vi "RT_Main.vi"() -> (2 "running":bool)   [LabVIEW 2018]
uses:
  <vilib>/FPGAPlugInAG/myRIO-1900/niLvFpga_Open_myRIO-1900.vi
  <vilib>/rvi/interface/common/dynamic/niFpgaDynamicAddResources.vi
  <vilib>/Utility/error.llb/Error Cluster From Error Code.vi
  <vilib>/rvi/errors/niLvFpgaAdjustHostInterfaceError.vi
  <vilib>/rvi/interface/common/niFpgaWaitOnOcc.vi
  <vilib>/FPGAPlugInAG/Dynamic/niLvFpga_Close_Dynamic.vi
  <vilib>/rvi/interface/nirviOpenFPGA/nirviOpenFPGA.xnode
  FPGA Bitfiles/FPGAPLL_FPGATarget_FPGAMain_V3ImA1lHnbc.lvbitx
  FPGA_Main.vi
  <vilib>/rvi/interface/nirviReadWriteControl/nirviReadWriteControl.xnode
  <vilib>/rvi/interface/nirviMethod/nirviMethod.xnode
  <vilib>/rvi/interface/nirviCloseFPGA/nirviCloseFPGA.xnode
  <vilib>/rvi/errors/niLvFpgaMergeErrorWithErrorCode.vi
  <vilib>/FPGAPlugInAG/Dynamic/niLvFpga_ReadFifo_Dynamic.vi
  <vilib>/FPGAPlugInAG/Dynamic/niLvFpga_ConfigureFifo_Dynamic.vi
  <vilib>/FPGAPlugInAG/Dynamic/niLvFpga_StartFifo_Dynamic.vi
  NiFpgaLv.dll
  <vilib>/rvi/interface/Simulation/niFpgaSimulationCallBeginRW.vi
panel:
  out "size(s)":i32
  out "error fifo\nread data":errorcluster
  out "#element left":u32
  out "#elements":u32
  out "error fifo start":errorcluster
  out "error fifo \ncheck #E":errorcluster
  out "error ref":errorcluster
  out "error closing":errorcluster
  out "error fifo config":errorcluster
  out "Actual Depth":u32
  # "RT Main"
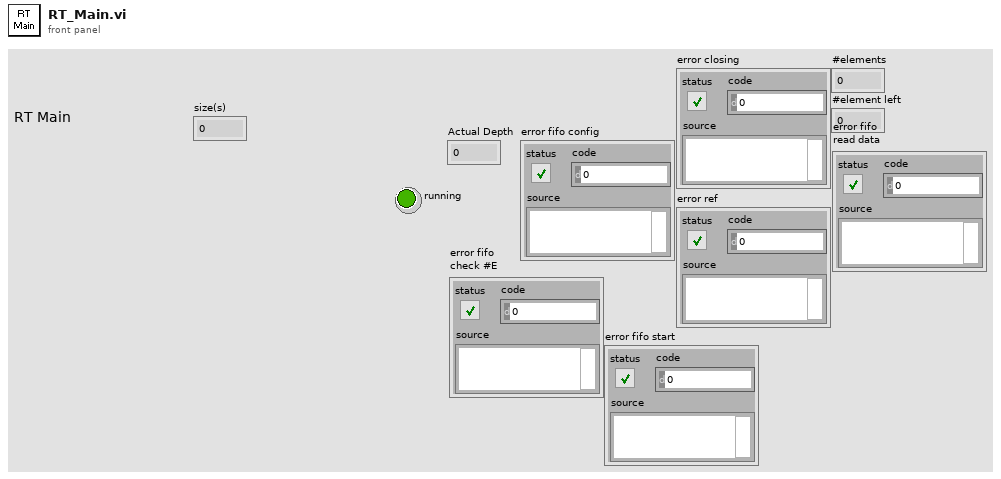
[diagram p1: front panel]
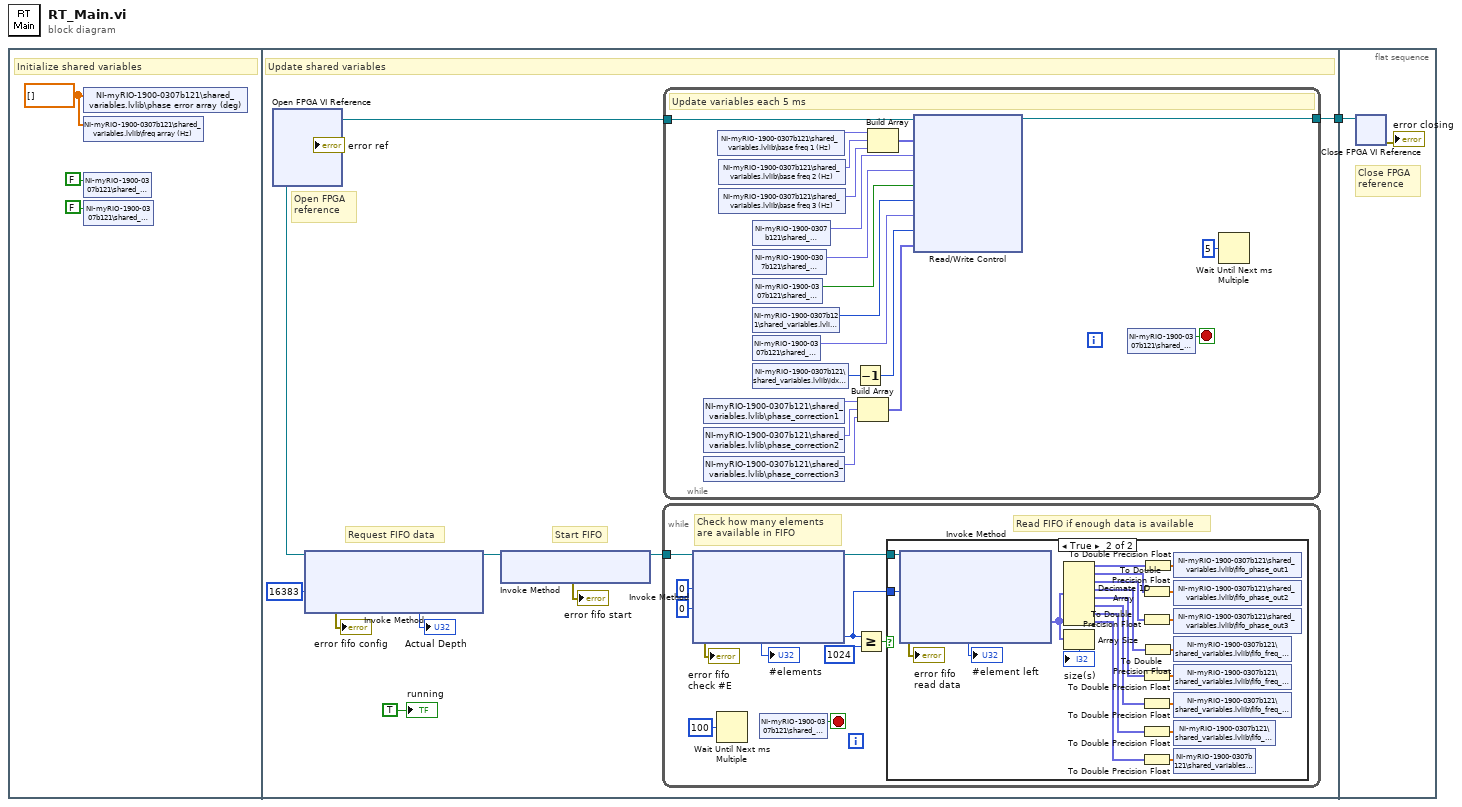
[diagram p0: block diagram]
diagram:
  n1 = flat-sequence {
    tunnel: [w13] -> w1
    tunnel: w1 -> [w67]
    frame #0 {
      w2 = dbl[] [] ("phase error array (deg)")
      # "Initialize shared variables"
      n2 = shared-variable "NI-myRIO-1900-0307b121\\shared_variables.lvlib\\phase error array (deg)"(w2) -> ()  [unwired: 1 in, 1 out]
      n3 = shared-variable "NI-myRIO-1900-0307b121\\shared_variables.lvlib\\freq array (Hz)"(w2) -> ()  [unwired: 1 in, 1 out]
      n4 = shared-variable "NI-myRIO-1900-0307b121\\shared_variables.lvlib\\stop"(FALSE ("stop")) -> ()  [unwired: 1 in, 1 out]
      n5 = shared-variable "NI-myRIO-1900-0307b121\\shared_variables.lvlib\\reset"(FALSE ("reset")) -> ()  [unwired: 1 in, 1 out]
    }
    frame #1 {
      # "Start FIFO"
      # "Request FIFO data"
      # "Open FPGA\nreference"
      # "Update shared variables"
      n6 = xnode "Open FPGA VI Reference"() -> ("FPGA VI Reference Out"=w12:refnum<k20>, "error out"=→"error ref":errorcluster)  [unwired: 2 in]
      n7 = xnode "Invoke Method"("FPGA VI Reference In"=w12, "Requested Depth"=u32 16383) -> ("FPGA VI Reference Out"=w7:refnum<k20>, "error out"=→"error fifo config":errorcluster, "Actual Depth"=→"Actual Depth":u32)  [unwired: 1 in]
      n8 = xnode "Invoke Method"("FPGA VI Reference In"=w7) -> ("FPGA VI Reference Out"=w5:refnum<k20>, "error out"=→"error fifo start":errorcluster)  [unwired: 1 in]
      n9 = while {
        tunnel: w5 -> [w23]
        stop <- w24 stop-if-true
        # "Read FIFO if enough data is available"
        # "Check how many elements\nare available in FIFO"
        n10 = xnode "Invoke Method"("FPGA VI Reference In"=w23, "Number of Elements"=u32 0, "Timeout (ms)"=0) -> ("FPGA VI Reference Out"=w18:refnum<k20>, "error out"=→"error fifo \ncheck #E":errorcluster, "Elements Remaining"=w16:u32)  [unwired: 1 in, 1 out]
        "#elements" <- w16
        n11 = Wait Until Next ms Multiple(millisecond multiple=u32 100) -> ()  [unwired: 1 out]
        n12 = shared-variable "NI-myRIO-1900-0307b121\\shared_variables.lvlib\\stop"() -> (w24:bool)  [unwired: 1 in, 1 out]
        n13 = Greater Or Equal?(x=w16, y=u32 1024) -> (x >= y?=w15:bool)
        n14 = case shown="True" w15 {
          tunnel: w18 -> [_ w46]
          tunnel: w16 -> [_ w41]
          frame False {
          }
          frame True {
            n15 = xnode "Invoke Method"("FPGA VI Reference In"=w46, "Number of Elements"=w41) -> ("error out"=→"error fifo\nread data":errorcluster, "Data"=w39:fxp<+/-,17,1>[], "Elements Remaining"=→"#element left":u32)  [unwired: 2 in, 1 out]
            n16 = Decimate 1D Array(w39) -> (w38:fxp<+/-,17,1>[], w37:fxp<+/-,17,1>[], w31:fxp<+/-,17,1>[], w30:fxp<+/-,17,1>[], w29:fxp<+/-,17,1>[], w28:fxp<+/-,17,1>[], w27:fxp<+/-,17,1>[], w25:fxp<+/-,17,1>[])
            n17 = Array Size(array=w39) -> (size(s)=→"size(s)":i32)
            n18 = To Double Precision Float(number=w37) -> (double precision float=w40:dbl[])
            n19 = To Double Precision Float(number=w31) -> (double precision float=w33:dbl[])
            n20 = To Double Precision Float(number=w29) -> (double precision float=w36:dbl[])
            n21 = To Double Precision Float(number=w28) -> (double precision float=w32:dbl[])
            n22 = To Double Precision Float(number=w27) -> (double precision float=w34:dbl[])
            n23 = To Double Precision Float(number=w25) -> (double precision float=w26:dbl[])
            n24 = To Double Precision Float(number=w38) -> (double precision float=w43:dbl[])
            n25 = To Double Precision Float(number=w30) -> (double precision float=w35:dbl[])
            n26 = shared-variable "NI-myRIO-1900-0307b121\\shared_variables.lvlib\\fifo_phase_out1"(w43) -> ()  [unwired: 1 in, 1 out]
            n27 = shared-variable "NI-myRIO-1900-0307b121\\shared_variables.lvlib\\fifo_phase_out2"(w40) -> ()  [unwired: 1 in, 1 out]
            n28 = shared-variable "NI-myRIO-1900-0307b121\\shared_variables.lvlib\\fifo_phase_out3"(w33) -> ()  [unwired: 1 in, 1 out]
            n29 = shared-variable "NI-myRIO-1900-0307b121\\shared_variables.lvlib\\fifo_freq_out1"(w35) -> ()  [unwired: 1 in, 1 out]
            n30 = shared-variable "NI-myRIO-1900-0307b121\\shared_variables.lvlib\\fifo_freq_out2"(w36) -> ()  [unwired: 1 in, 1 out]
            n31 = shared-variable "NI-myRIO-1900-0307b121\\shared_variables.lvlib\\fifo_freq_out3"(w32) -> ()  [unwired: 1 in, 1 out]
            n32 = shared-variable "NI-myRIO-1900-0307b121\\shared_variables.lvlib\\fifo_adc_in"(w34) -> ()  [unwired: 1 in, 1 out]
            n33 = shared-variable "NI-myRIO-1900-0307b121\\shared_variables.lvlib\\fifo_ref"(w26) -> ()  [unwired: 1 in, 1 out]
          }
        }
      }
      n34 = while {
        tunnel: w12 -> [w65]
        tunnel: [w60] -> w13
        stop <- w59 stop-if-true
        # "Update variables each 5 ms"
        n35 = shared-variable "NI-myRIO-1900-0307b121\\shared_variables.lvlib\\phase_correction1"() -> (w50:fxp<+/-,64,32>)  [unwired: 1 in, 1 out]
        n36 = shared-variable "NI-myRIO-1900-0307b121\\shared_variables.lvlib\\phase_correction2"() -> (w49:fxp<+/-,64,32>)  [unwired: 1 in, 1 out]
        n37 = shared-variable "NI-myRIO-1900-0307b121\\shared_variables.lvlib\\phase_correction3"() -> (w48:fxp<+/-,64,32>)  [unwired: 1 in, 1 out]
        n38 = shared-variable "NI-myRIO-1900-0307b121\\shared_variables.lvlib\\base freq 1 (Hz)"() -> (w56:fxp<+/-,64,32>)  [unwired: 1 in, 1 out]
        n39 = shared-variable "NI-myRIO-1900-0307b121\\shared_variables.lvlib\\base freq 2 (Hz)"() -> (w55:fxp<+/-,64,32>)  [unwired: 1 in, 1 out]
        n40 = shared-variable "NI-myRIO-1900-0307b121\\shared_variables.lvlib\\base freq 3 (Hz)"() -> (w53:fxp<+/-,64,32>)  [unwired: 1 in, 1 out]
        n41 = shared-variable "NI-myRIO-1900-0307b121\\shared_variables.lvlib\\P gain"() -> (w63:fxp<+/-,64,32>)  [unwired: 1 in, 1 out]
        n42 = shared-variable "NI-myRIO-1900-0307b121\\shared_variables.lvlib\\I gain"() -> (w62:fxp<+/-,64,32>)  [unwired: 1 in, 1 out]
        n43 = shared-variable "NI-myRIO-1900-0307b121\\shared_variables.lvlib\\reset"() -> (w61:bool)  [unwired: 1 in, 1 out]
        n44 = shared-variable "NI-myRIO-1900-0307b121\\shared_variables.lvlib\\idx_pick"() -> (w58:u8)  [unwired: 1 in, 1 out]
        n45 = shared-variable "NI-myRIO-1900-0307b121\\shared_variables.lvlib\\gain"() -> (w54:fxp<+,20,8>)  [unwired: 1 in, 1 out]
        n46 = shared-variable "NI-myRIO-1900-0307b121\\shared_variables.lvlib\\idx_scope"() -> (w52:u8)  [unwired: 1 in, 1 out]
        n47 = Decrement(x=w52) -> (x-1=w51:u8)
        n48 = Build Array(w50, w49, w48) -> (w47:fxp<+/-,64,32>[])
        n49 = Build Array(w56, w55, w53) -> (w57:fxp<+/-,64,32>[])
        n50 = xnode "Read/Write Control"("FPGA VI Reference In"=w65, "base freqs"=w57, "P gain"=w63, "I gain"=w62, "reset"=w61, "idx pick"=w58, "gain"=w54, "idx scope"=w51, "phase_correction"=w47) -> ("FPGA VI Reference Out"=w60:refnum<k20>)  [unwired: 1 in, 1 out]
        n51 = shared-variable "NI-myRIO-1900-0307b121\\shared_variables.lvlib\\stop"() -> (w59:bool)  [unwired: 1 in, 1 out]
        n52 = Wait Until Next ms Multiple(millisecond multiple=u32 5) -> ()  [unwired: 1 out]
      }
      "running" <- TRUE ("running")
    }
    frame #2 {
      # "Close FPGA\nreference"
      n53 = xnode "Close FPGA VI Reference"("FPGA VI Reference In"=w67) -> ("error out"=→"error closing":errorcluster)  [unwired: 1 in]
    }
  }
